vi "Read Package.vi"(8 "error in (no error)":errorcluster, 11 "Test Suite in":refnum<class "Test Suite.lvclass">) -> (0 "error out":errorcluster, 2 "Package":string, 3 "Test Suite out":refnum<class "Test Suite.lvclass">)   [LabVIEW 2013, in "JUnit XML.lvlib" / "Test Suite.lvclass"]
uses:
  Test Suite.lvclass
  Test Suite.lvclass/Test Suite.ctl
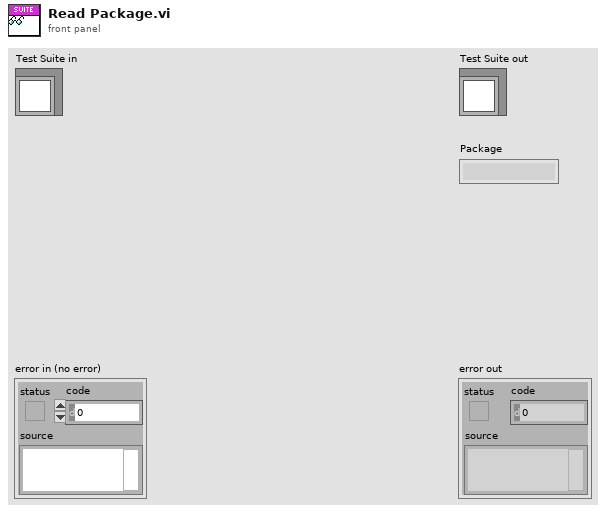
[diagram p1: front panel]
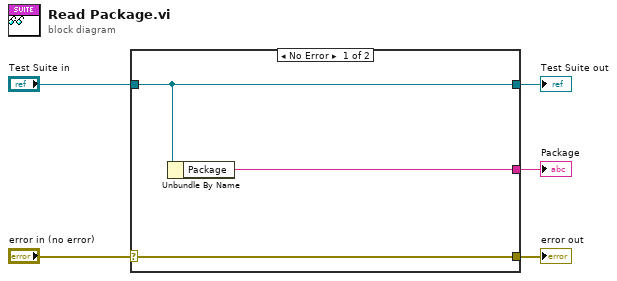
[diagram p0: block diagram]
diagram:
  n1 = case shown="No Error" "error in (no error)" {
    selector: "error in (no error)" -> [w8 w9]
    tunnel: [w8 w9] -> w4
    tunnel: [w7 w10] -> w2
    tunnel: "Test Suite in" -> [w7 w10]
    tunnel: [w6 _] -> w1
    frame No Error {
      n2 = Unbundle By Name(w7) -> ("Package"=w6:string)
    }
    frame Error {
    }
  }
  "error out" <- w4
  "Test Suite out" <- w2
  "Package" <- w1
